vi "ReplaceTextFile.vi"(9 "file path (use dialog)":path, 10 "Boolean":bool, 11 "String":string) -> ()   [LabVIEW 2014]
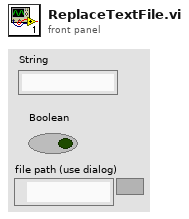
[diagram p1: front panel]
types:
  T1 = enum16{"open", "replace", "create", "open or create", "replace or create", "replace or create with confirmation"}
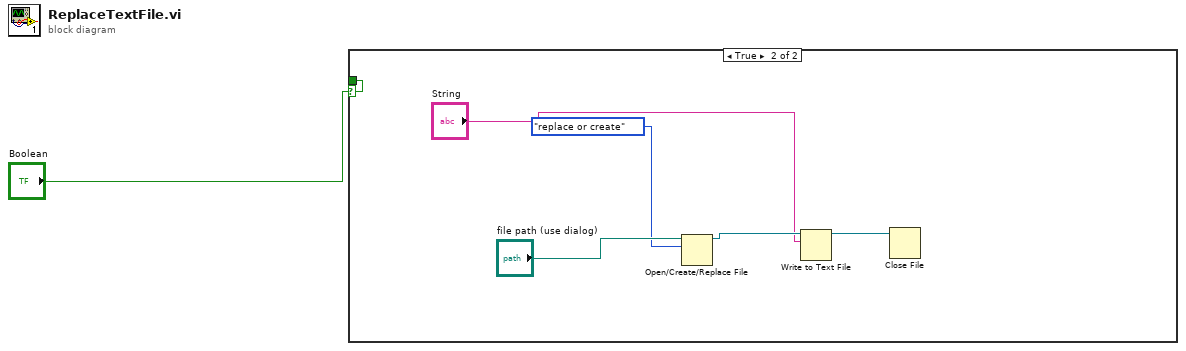
[diagram p0: block diagram]
diagram:
  n1 = case shown="True" "Boolean" {
    selector: "Boolean" -> [w2 w8]
    tunnel: [w2 w8] -> _
    frame False {
    }
    frame True {
      n2 = Open/Create/Replace File(file path (use dialog)="file path (use dialog)", operation (0:open)=T1."replace or create") -> (refnum out=w5:refnum<file>)  [unwired: 4 in, 2 out]
      n3 = Write to Text File(file (use dialog)=w5, text="String") -> (refnum out=w6:refnum<file>)  [unwired: 2 in, 2 out]
      n4 = Close File(refnum=w6) -> ()  [unwired: 1 in, 2 out]
    }
  }
